vi "TagDB Refmgr-Reset.vi"(8 "error in (no error)":errorcluster, 10 "RegExp":string, 11 "TagDB in":T1) -> (0 "error out":errorcluster, 1 "Keys":string[](array[string]), 3 "TagDB out":T1)   [LabVIEW 2017, in "TagDB RefManager.lvlib"]
uses:
  TagDB RefManager.lvlib
  <userlib>/_NEVSTOP/TagDB/Typedef/TagDB.ctl
  d0e574de-2f92-4d87-b90b-b90933c7e763.vi
  <userlib>/_NEVSTOP/TagDB/_Support/Error/_Clear Errors.vi
  d0e574de-2f92-4d87-b90b-b90933c7e763.vi/29b2ea6d-6d7f-4e4a-ad31-a5cb760462c7.vi
  <userlib>/_NEVSTOP/TagDB/API/TagDB-Status.vi
  <userlib>/_NEVSTOP/TagDB/_Support/DataAccess/_NameCacher.vi
  <userlib>/_NEVSTOP/TagDB/_Support/Change Detector/TagDB dbChanged.vi
  <userlib>/_NEVSTOP/TagDB/_Support/DataAccess/TagDB Ref to DVR.vi
  <userlib>/_NEVSTOP/TagDB/_Support/Error/_[error50000]Invalid DB REF.vi
  <userlib>/_NEVSTOP/TagDB/_Support/URL/TRIM-BOTH-SPACE.vi
  <userlib>/_NEVSTOP/TagDB/_Support/Error/_[error50002]Invalid DataType.vi
  <userlib>/_NEVSTOP/TagDB/TagDB.lvlib
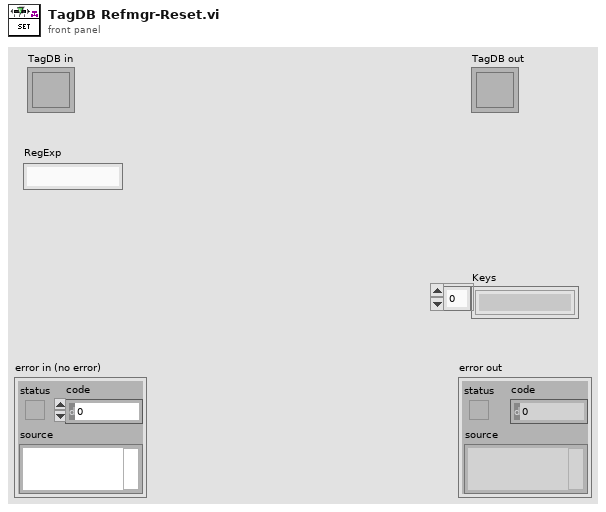
[diagram p1: front panel]
types:
  T1 = typedef "TagDB.lvlib/TagDB.ctl" = refnum<k1>
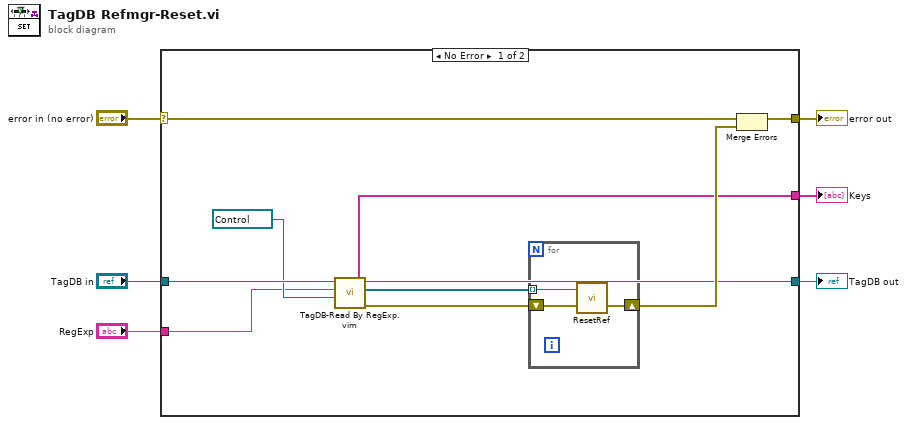
[diagram p0: block diagram]
diagram:
  n1 = case shown="No Error" "error in (no error)" {
    selector: "error in (no error)" -> [w15 w21]
    tunnel: [w16 w21] -> w6
    tunnel: "TagDB in" -> [w13 w20]
    tunnel: "RegExp" -> [w11 _]
    tunnel: [w7 _] -> w2
    tunnel: [w8 w20] -> w1
    frame No Error {
      n2 = call "TagDB-Read By RegExp.vim"("Type"=refnum<vi> refnum, "RegExp"=w11, "DB Ref"=w13) -> ("error out"=w9:errorcluster, "names"=w7:string[], "value"=w10:refnum<vi>[], "DB Ref(dup)"=w8:T1)  [unwired: 5 in]
      n3 = for {
        tunnel: w10 -> [w19] mode=indexing
        shift-right: [w17] -> w14
        shift-left: w9 -> [w18]
        n4 = call "ResetRef.vi"("error in (no error)"=w18, "Boolean in"=w19) -> ("error out"=w17:errorcluster)  [unwired: 8 in, 1 out]
      }
      n5 = Merge Errors(w15, w14) -> (w16:errorcluster)
    }
    frame Error {
    }
  }
  "error out" <- w6
  "TagDB out" <- w1
  "Keys" <- w2
